vi "Read Min Max Waveform.vi"(8 "error in (no error)":errorcluster, 9 "Timeout (10000 ms)":u32=10000, 10 "Source (0: Channel 1)":u16(ring) items=["Channel 1", "Channel 2", "Channel 3", "Channel 4", "Math"], 11 "VISA resource name":refnum<visa-resource-name>) -> (0 "error out":errorcluster, 1 "Min Waveform":waveform(dbl)(graph), 2 "Max Waveform":waveform(dbl)(graph), 3 "VISA resource name out":refnum<visa-resource-name>)   [LabVIEW 2018, in "Agilent 6000 Series.lvlib"]
doc: "Initiates an acquisition on all channels that you enabled with the <B>Configure Channel</B> VI. The VI waits for the acquisition to complete and returns the minimum and maximum waveforms for the Source channel you specified. If the oscilloscope did not complete the acquisition within the time period you specify with the Timeout parameter, the VI returns a time out error. A common cause for a timeout error is the acquisition was not triggered. For example, the trigger level is out of range of the waveform.\n\nCall the <B>Fetch Min Max Waveform</B> VI to obtain the waveforms for each of the remaining enabled Source channels without initiating another acquisition.\n\n<B>NOTE:</B>\n\n1. This VI should ONLY be used when Acquisition Type is Peak Detect.\n\n2. If your instrument does not support auto compensation for probe attenuation, you may need to adjust the scaling of the Waveform Data accordingly. This is handled automatically in the <B>Configure Channel</B> VI or can be done manually by multiplying the Waveform Data by the probe attenuation."
uses:
  Agilent 6000 Series.lvlib
  Low Data VIs/Fetch Min Max Waveform.vi
panel:
  # "NOTE: This VI should ONLY be used when Acquisition Type is Peak Detect"
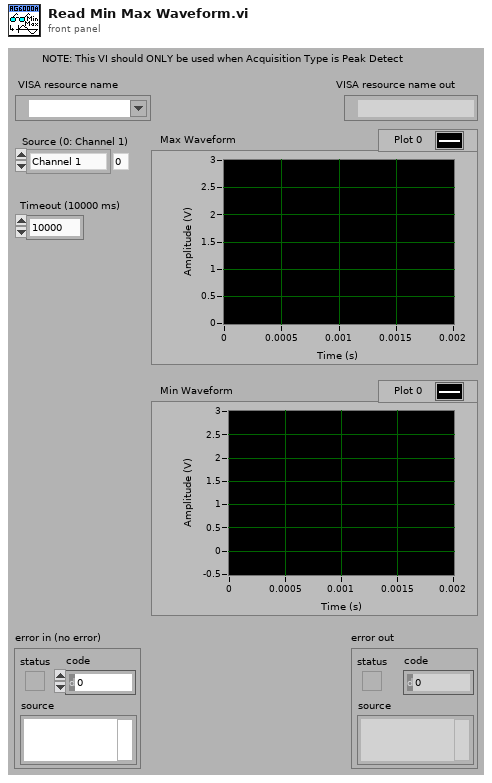
[diagram p1: front panel]
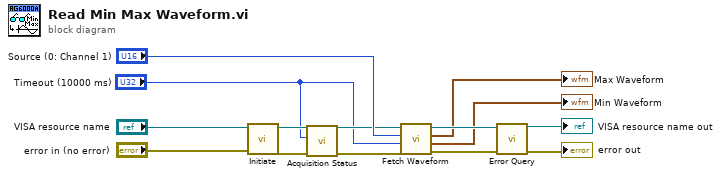
[diagram p0: block diagram]
diagram:
  n1 = call "Initiate.vi"("error in (no error)"="error in (no error)", "VISA resource name"="VISA resource name") -> ("error out"=w6:errorcluster, "VISA resource name out"=w7:refnum<visa-resource-name>)  [unwired: 8 in]
  n2 = call "Acquisition Status.vi"("error in (no error)"=w6, "Timeout (10000 ms)"="Timeout (10000 ms)", "VISA resource name"=w7) -> ("error out"=w5:errorcluster, "VISA resource name out"=w4:refnum<visa-resource-name>)  [unwired: 6 in, 1 out]
  n3 = call-poly "Fetch Waveform.vi"("error in (no error)"=w5, "Timeout (10000 ms)"="Timeout (10000 ms)", "Source (0: Channel 1)"="Source (0: Channel 1)", "VISA resource name"=w4) -> ("error out"=w9:errorcluster, "Min Waveform"=→"Min Waveform":waveform(dbl), "Max Waveform"=→"Max Waveform":waveform(dbl), "VISA resource name out"=w10:refnum<visa-resource-name>)  [unwired: 4 in]
  n4 = call "Error Query.vi"("error in (no error)"=w9, "VISA resource name"=w10) -> ("error out"=→"error out":errorcluster, "VISA resource name out"=→"VISA resource name out":refnum<visa-resource-name>)  [unwired: 6 in, 2 out]
